vi "CheckForExistingErrorControl.vi"(8 "error in (no error)":errorcluster, 11 "Control terminals to check":refnum<vi>[](array[refnum])) -> (0 "error out":errorcluster, 2 "Error control ref":refnum<vi>, 3 "Error control found?":bool)   [LabVIEW 2017, in "ErrorStructureDrawer.lvlib"]
doc: "Checks if the input array of control terminal references contains any references to an error cluster (i.e. to an error control or error indicator). If so, returns a \"true\" boolean, and also the first corresponding reference found."
uses:
  ErrorStructureDrawer.lvlib
  <vilib>/Utility/Data Type/Type Definitions/Data Type.ctl
  <vilib>/Utility/Data Type/NI_Data Type.lvlib
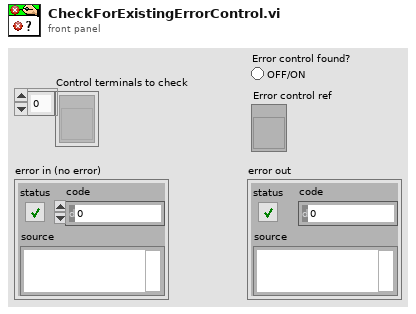
[diagram p1: front panel]
types:
  T1 = typedef "NI_Data Type.lvlib/Data Type.ctl" = enum8{"Invalid Type", "Void", "I8", "I16", "I32", "I64", "U8", "U16", "U32", "U64", "Single Float", "Double Float", "Extended Float", "Single Complex", "Double Complex", "Extended Complex", "Enum U8", "Enum U16", "Enum U32", "Enum U64", "Single Float With Unit", "Double Float With Unit", "Extended Float With Unit", "Single Complex with Unit", "Double Complex with Unit", "Extended Complex with Unit", "Boolean", "String", "Path", "Picture", "Tag", "Array", "Cluster", "Variant", "LV Variant", "Waveform", "Timestamp", "Digital Waveform", "Digital Data", "ExpressData", "Refnum", "External Data", "VI", "Poly VI", "LabVIEW Class Instance", "Fixed Point"}
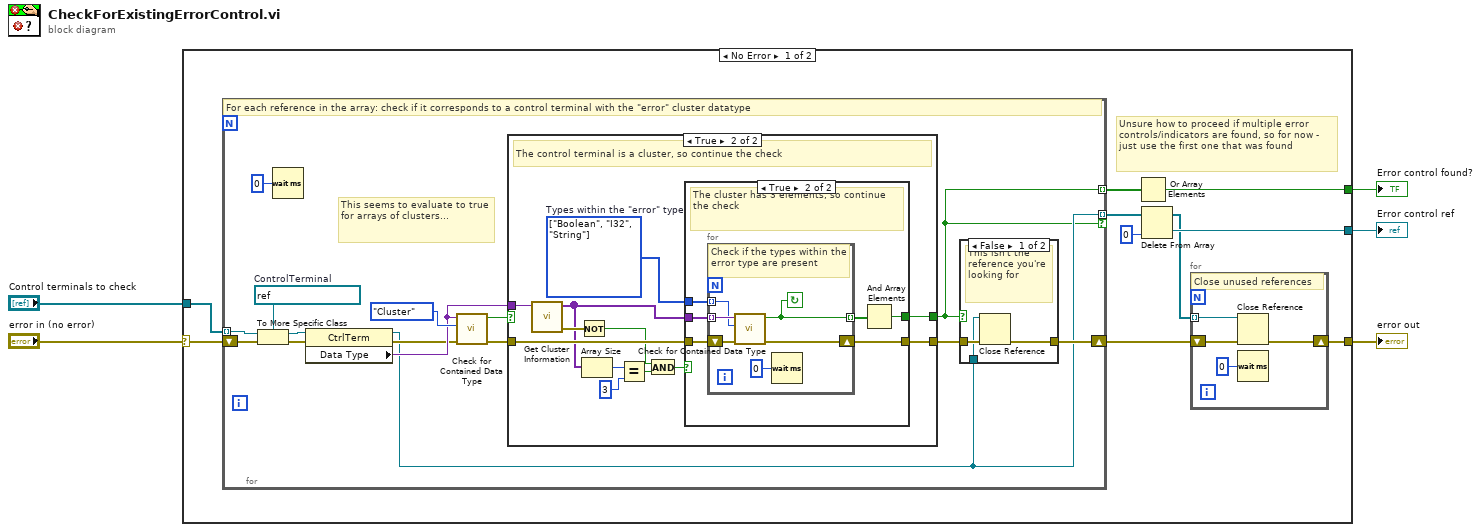
[diagram p0: block diagram]
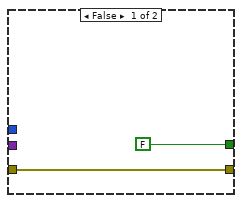
[diagram p4: hidden frame]
diagram:
  n1 = case shown="No Error" "error in (no error)" {
    selector: "error in (no error)" -> [w10 w66]
    tunnel: "Control terminals to check" -> [w15 _]
    tunnel: [w11 w66] -> w4
    tunnel: [w9 _] -> w2
    tunnel: [w6 _] -> w1
    frame No Error {
      # "Unsure how to proceed if multiple error controls/indicators are found, so for now - just use the first one that was found"
      n2 = for {
        tunnel: w15 -> [w34] mode=indexing
        shift-right: [w22] -> w12
        shift-left: w10 -> [w31]
        tunnel: [w21] -> w14 mode=indexing if=w20
        tunnel: [w20] -> w7 mode=indexing
        w32 = refnum<vi> refnum  # ControlTerminal
        # "This seems to evaluate to true for arrays of clusters..."
        # "For each reference in the array: check if it corresponds to a control terminal with the \"error\" cluster datatype"
        n3 = To More Specific Class(target class=w32, reference=w34, error in=w31) -> (specific class reference=w33:refnum<vi>, error out=w30:errorcluster)
        n4 = Wait (ms)(milliseconds to wait=u32 0) -> ()  [unwired: 1 out]
        n5 = property class="CtrlTerm"(reference=w33, error in=w30) -> (reference out=w21:refnum<vi>, error out=w24:errorcluster, "Data Type"=w26:variant)
        n6 = call <vilib>:"Check for Contained Data Type.vi"("error in (no error)"=w24, "Data Type to Find"=Data_Type."Cluster", "Variant"=w26) -> ("error out"=w28:errorcluster, "Contains Data Type to Find?"=w27:bool)  [unwired: 7 in]
        n7 = case shown="True" w27 {
          tunnel: w28 -> [w39 w46]
          tunnel: [w39 w49] -> w23
          tunnel: w26 -> [_ w51]
          tunnel: [_ w47] -> w20
          frame False {
          }
          frame True {
            w48 = T1[] [enum."Boolean", enum."I32", enum."String"] items=["Invalid Type", "Void", "I8", "I16", "I32", "I64", "U8", "U16", "U32", "U64", "Single Float", "Double Float", "Extended Float", "Single Complex", "Double Complex", "Extended Complex", "Enum U8", "Enum U16", "Enum U32", "Enum U64", "Single Float With Unit", "Double Float With Unit", "Extended Float With Unit", "Single Complex with Unit", "Double Complex with Unit", "Extended Complex with Unit", "Boolean", "String", "Path", "Picture", "Tag", "Array", "Cluster", "Variant", "LV Variant", "Waveform", "Timestamp", "Digital Waveform", "Digital Data", "ExpressData", "Refnum", "External Data", "VI", "Poly VI", "LabVIEW Class Instance", "Fixed Point"]  # Types within the "error" type
            # "The control terminal is a cluster, so continue the check"
            n8 = call <vilib>:"Get Cluster Information.vi"("Variant"=w51) -> ("error out"=w44:errorcluster, "Cluster Elements"=w43:variant[])  [unwired: 9 in]
            n9 = Not(x=w44) -> (.not. x?=w41:bool)
            n10 = Array Size(array=w43) -> (size(s)=w45:i32)
            n11 = Equal?(x=w45, y=3) -> (x = y?=w42:bool)
            n12 = And(x=w41, y=w42) -> (x .and. y?=w40:bool)
            n13 = case shown="True" w40 {
              tunnel: [w53 w57] -> w49
              tunnel: w46 -> [w53 w59]
              tunnel: w43 -> [_ w58]
              tunnel: [FALSE w55] -> w47
              tunnel: w48 -> [_ w54]
              frame False {
              }
              frame True {
                # "The cluster has 3 elements, so continue the check"
                n14 = for {
                  shift-right: [w63] -> w57
                  shift-left: w59 -> [w65]
                  tunnel: w58 -> [w64] mode=indexing
                  tunnel: [w60] -> w56 mode=indexing
                  tunnel: w54 -> [w62] mode=indexing
                  stop <- w60 continue-if-true
                  # "Check if the types within the error type are present"
                  n15 = call <vilib>:"Check for Contained Data Type.vi"("error in (no error)"=w65, "Data Type to Find"=w62, "Variant"=w64) -> ("error out"=w63:errorcluster, "Contains Data Type to Find?"=w60:bool)  [unwired: 7 in]
                  n16 = Wait (ms)(milliseconds to wait=u32 0) -> ()  [unwired: 1 out]
                }
                n17 = And Array Elements(Boolean array=w56) -> (logical AND=w55:bool)
              }
            }
          }
        }
        n18 = case shown="False" w20 {
          tunnel: w23 -> [w37 w38]
          tunnel: [w36 w38] -> w22
          tunnel: w21 -> [w35 _]
          frame False {
            # "This isn't the reference you're looking for"
            n19 = Close Reference(reference=w35, error in (no error)=w37) -> (error out=w36:errorcluster)
          }
          frame True {
            # "Reference is an error cluster, so don't close it"
          }
        }
      }
      n20 = Or Array Elements(Boolean array=w7) -> (logical OR=w6:bool)
      n21 = Delete From Array(array=w14, index=0) -> (deleted portion=w9:refnum<vi>, array with subset deleted=w8:refnum<vi>[])  [unwired: 1 in]
      n22 = for {
        tunnel: w8 -> [w19] mode=indexing
        shift-right: [w17] -> w11
        shift-left: w12 -> [w18]
        # "Close unused references"
        n23 = Close Reference(reference=w19, error in (no error)=w18) -> (error out=w17:errorcluster)
        n24 = Wait (ms)(milliseconds to wait=u32 0) -> ()  [unwired: 1 out]
      }
    }
    frame Error {
    }
  }
  "error out" <- w4
  "Error control ref" <- w2
  "Error control found?" <- w1
